vi "nano-positioner.vi"() -> ()   [LabVIEW 2014]
uses:
  <vilib>/Utility/inputDevices.llb/keyboardAcquire.vi
  <userlib>/Madlib/Madlib.dll
panel:
  in  "?":bool
  in  "Motion Multiplier":dbl(slide)=1.0 scale=1.0..100.0
  in  "Command rate":u16(ring)=10 items=["500 Hertz"=2, "100 Hertz"=10, "10 Hertz"=100, "1 Hertz"=1000]
  out "First Key":T1(ring)
  in  "Max Velocity":string(combo)="22"
  in  "Z Decreasing":string(combo)="21"
  in  "Z Increasing":string(combo)="24"
  in  "X Increasing":string(combo)="32"
  in  "X Decreasing":string(combo)="28"
  in  "Y Decreasing":string(combo)="10"
  in  "Y Increasing":string(combo)="13"
  out "Z (mM)":dbl format="%#_13g"
  out "Y (mM)":dbl format="%#_13g"
  out "X (mM)":dbl format="%#_13g"
  out "Z Range (mM)":dbl format="%#_13g"
  out "Y Range (mM)":dbl format="%#_13g"
  out "X Range (mM)":dbl format="%#_13g"
  # "Key Configuration"
  # "Command Rate"
  # "Motion Multiplier"
  # "x1"
  # "x100"
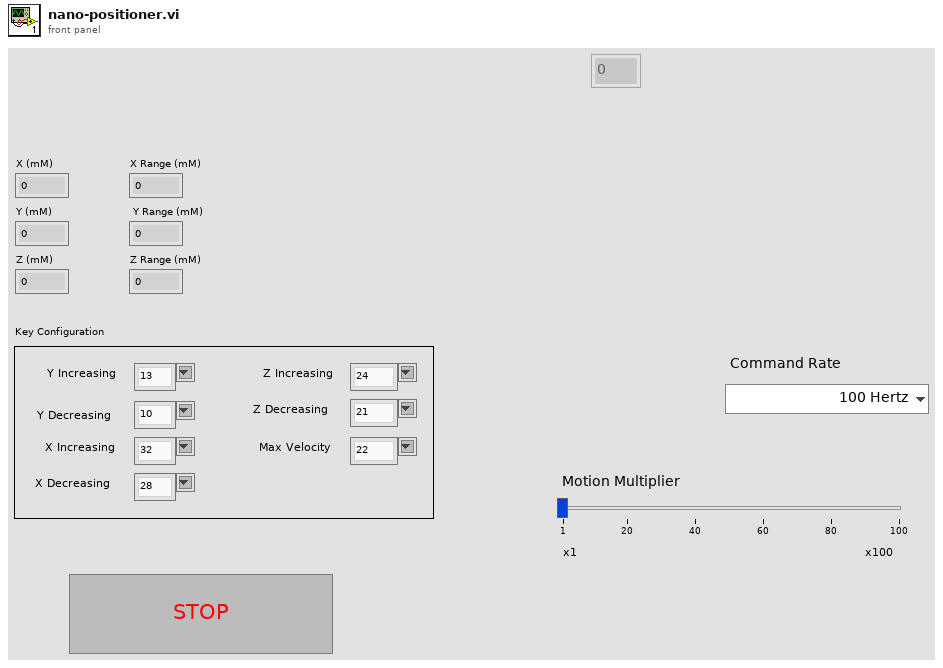
[diagram p1: front panel]
types:
  T1 = enum16{"0", "1", "2", "3", "4", "5", "6", "7", "8", "9", "A", "B", "C", "D", "E", "F", "G", "H", "I", "J", "K", "L", "M", "N", "O", "P", "Q", "R", "S", "T", "U", "V", "W", "X", "Y", "Z", "F1", "F2", "F3", "F4", "F5", "F6", "F7", "F8", "F9", "F10", "F11", "F12", "F13", "F14", "F15", "ADD", "BACK", "BACKSLASH", "CAPITAL", "COMMA", "DECIMAL", "DELETE", "DIVIDE", "DOWN", "END", "EQUALS", "ESCAPE", "GRAVE (`)", "HOME", "INSERT", "LBRACKET", "LCONTROL", "LEFT", "L ALT", "LSHIFT", "LWIN", "MINUS", "MULTIPLY", "NEXT", "NUMLOCK", "NUMPAD_0", "NUMPAD_1", "NUMPAD_2", "NUMPAD_3", "NUMPAD_4", "NUMPAD_5", "NUMPAD_6", "NUMPAD_7", "NUMPAD_8", "NUMPAD_9", "PAUSE", "PERIOD", "PRIOR (PG UP)", "RBRACKET", "RCONTROL", "RETURN", "RIGHT", "R ALT", "RSHIFT", "RWIN", "SCROLL", "SEMICOLON", "SLASH", "SPACE", "SUBTRACT", "TAB", "UP", "ENTER (num pad)", "' (quote)"}
  T2 = cluster{"X Command":dbl, "Y Command":dbl, "Z Command":dbl, "X Position":dbl, "Y Position":dbl, "Z Position":dbl, "X Calibration":dbl, "Y Calibration":dbl, "Z Calibration":dbl}
  T3 = cluster{"X Command":dbl, "Y Command":dbl, "Z Command":dbl, "X Position":dbl, "Y Position":dbl, "Z Position":dbl}
  T4 = enum16{"0", "1", "2", "3", "4", "5", "6", "7", "8", "9", "A", "B", "C", "D", "E", "F", "G", "H", "I", "J", "K", "L", "M", "N", "O", "P", "Q", "R", "S", "T", "U", "V", "W", "X", "Y", "Z", "F1", "F2", "F3", "F4", "F5", "F6", "F7", "F8", "F9", "F10", "F11", "F12", "F13", "F14", "F15", "ADD", "BACK", "BACKSLASH", "CAPITAL", "COMMA", "DECIMAL", "DELETE", "DIVIDE", "DOWN", "END", "EQUALS", "ESCAPE", "GRAVE (`)", "HOME", "INSERT", "LBRACKET", "LCONTROL", "LEFT", "L ALT", "LSHIFT", "LWIN", "MINUS", "MULTIPLY", "NEXT", "NUMLOCK", "NUMPAD_0", "NUMPAD_1", "NUMPAD_2", "NUMPAD_3", "NUMPAD_4", "NUMPAD_5", "NUMPAD_6", "NUMPAD_7", "NUMPAD_8", "NUMPAD_9", "PAUSE", "PERIOD", "PRIOR (PG UP)", "RBRACKET", "RCONTROL", "RETURN", "RIGHT", "R ALT", "RSHIFT", "RWIN", "SCROLL", "SEMICOLON", "SLASH", "SPACE", "SUBTRACT", "TAB", "UP", "ENTER (num pad)", "' (quote)"}[]
  T5 = cluster{"Y Increasing":string, "Y Decreasing":string, "X Increasing":string, "X Decreasing":string, "Z Increasing":string, "Z Decreasing":string, "Max Velocity":string}
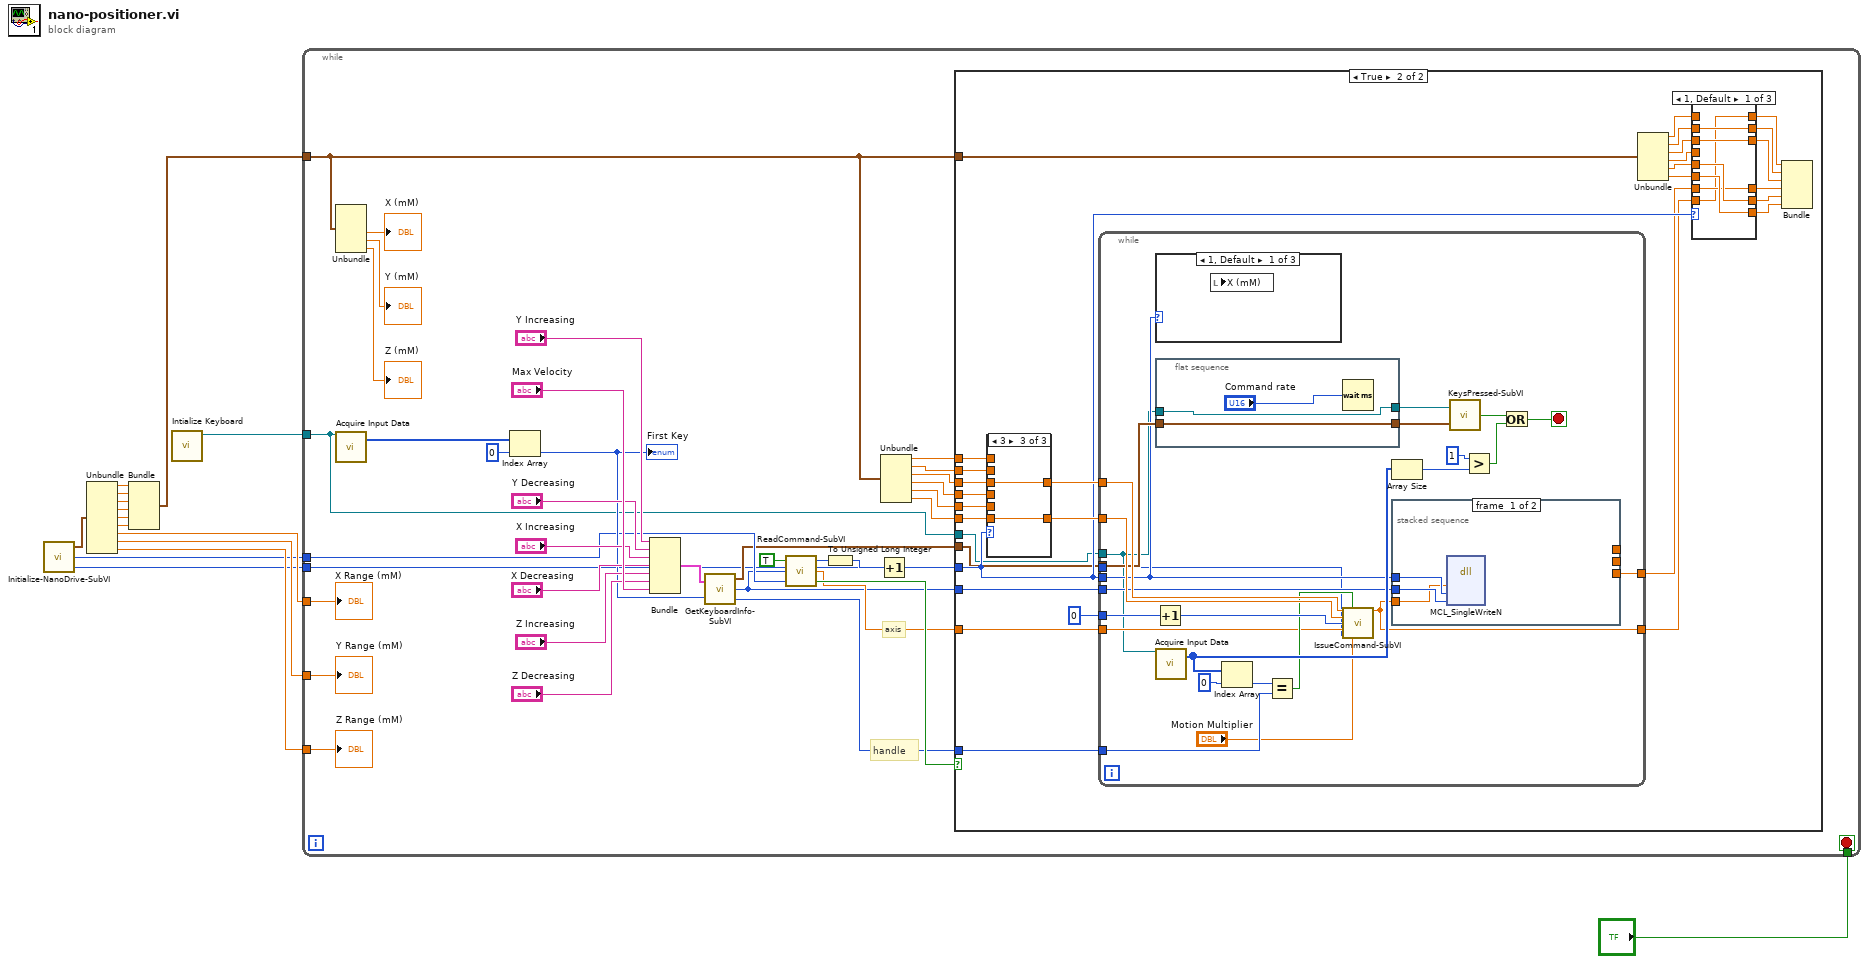
[diagram p0: block diagram]
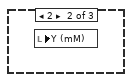
[diagram p5: hidden frame]
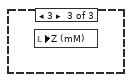
[diagram p6: hidden frame]
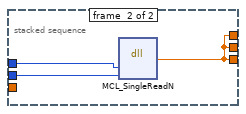
[diagram p7: hidden frame]
diagram:
  n1 = call <userlib>:"Initialize-NanoDrive-SubVI.vi"() -> ("Output Pos Info"=w15:T2, "Handle"=w3:i32, "ADC/DAC Resolution"=w2:u32)  [unwired: 1 in]
  n2 = Unbundle(w15) -> ("X Command"=w11:dbl, "Y Command"=w10:dbl, "Z Command"=w9:dbl, "X Position"=w8:dbl, "Y Position"=w7:dbl, "Z Position"=w6:dbl, "X Calibration"=w14:dbl, "Y Calibration"=w13:dbl, "Z Calibration"=w12:dbl)
  n3 = Bundle("X Command"=w11, "Y Command"=w10, "Z Command"=w9, "X Position"=w8, "Y Position"=w7, "Z Position"=w6) -> (w5:T3)  [unwired: 1 in]
  n4 = call <vilib>:"Intialize Keyboard.vi"() -> ("device ID"=w4:refnum<k1>)  [unwired: 1 in, 10 out]
  n5 = while {
    tunnel: w14 -> [w52]
    tunnel: w13 -> [w51]
    tunnel: w12 -> [w50]
    tunnel: w5 -> [w46]
    tunnel: w4 -> [w19]
    tunnel: w3 -> [w33]
    tunnel: w2 -> [w17]
    tunnel: "?" -> [w16]
    stop <- w16 stop-if-true
    # "handle"
    # "axis"
    n6 = Unbundle(w46) -> ("X Position"=→"X (mM)":dbl, "Y Position"=→"Y (mM)":dbl, "Z Position"=→"Z (mM)":dbl)  [unwired: 3 out]
    n7 = call-poly <vilib>:"Acquire Input Data.vi"("device ID"=w19) -> ("keys pressed"=w37:T4)  [unwired: 1 in, 17 out]
    n8 = Index Array "Index Array"(array=w37, index=0) -> (element=w35:T1)
    "First Key" <- w35
    n9 = Bundle("Y Increasing"="Y Increasing", "Y Decreasing"="Y Decreasing", "X Increasing"="X Increasing", "X Decreasing"="X Decreasing", "Z Increasing"="Z Increasing", "Z Decreasing"="Z Decreasing", "Max Velocity"="Max Velocity") -> (w38:T5)  [unwired: 1 in]
    n10 = call <userlib>:"GetKeyboardInfo-SubVI.vi"("Key Selections"=w38, "Key\nValue"=w35) -> ("Key values"=w20:cluster{i32, i32, i32, i32, i32, i32, i32}, "number"=w18:u32, "Max Velocity Value"=w22:i32)
    n11 = call <userlib>:"ReadCommand-SubVI.vi"("handle"=w33, "Motion #"=w18, "Enable\n(True)"=TRUE) -> ("Enable Move\n(TRUE)"=w32:bool, "Direction"=w21:dbl, "Axis"=w31:enum16{"X", "Y", "Z"})
    n12 = To Unsigned Long Integer(number=w31) -> (unsigned 32bit integer=w30:u32)
    n13 = Increment(x=w30) -> (x+1=w29:u32)
    n14 = Unbundle(w46) -> ("X Command"=w27:dbl, "Y Command"=w26:dbl, "Z Command"=w24:dbl, "X Position"=w28:dbl, "Y Position"=w25:dbl, "Z Position"=w23:dbl)
    n15 = case shown="True" w32 {
      tunnel: w46 -> [_ w83]
      tunnel: w29 -> [_ w61]
      tunnel: w28 -> [_ w82]
      tunnel: w27 -> [_ w81]
      tunnel: w26 -> [_ w78]
      tunnel: w25 -> [_ w77]
      tunnel: w24 -> [_ w76]
      tunnel: w23 -> [_ w75]
      tunnel: w22 -> [_ w60]
      tunnel: w21 -> [_ w59]
      tunnel: w20 -> [_ w58]
      tunnel: w19 -> [_ w57]
      tunnel: w18 -> [_ w56]
      tunnel: w17 -> [_ w53]
      frame False {
      }
      frame True {
        n16 = case shown="3" w61 {
          tunnel: [w85 w86 w88] -> w79
          tunnel: w82 -> [w85 _ _]
          tunnel: w81 -> [w84 _ _]
          tunnel: [w84 w87 w89] -> w80
          tunnel: w78 -> [_ w87 _]
          tunnel: w77 -> [_ w86 _]
          tunnel: w76 -> [_ _ w89]
          tunnel: w75 -> [_ _ w88]
          frame 1, Default {
          }
          frame 2 {
          }
          frame 3 {
          }
        }
        n17 = while {
          tunnel: w80 -> [w114]
          tunnel: w79 -> [w113]
          tunnel: 0 -> [w112]
          tunnel: w61 -> [w94]
          tunnel: w60 -> [w106]
          tunnel: w59 -> [w105]
          tunnel: w58 -> [w102]
          tunnel: w57 -> [w91]
          tunnel: w56 -> [w95]
          tunnel: [w93] -> w55
          tunnel: [w92] -> w54
          tunnel: w53 -> [w90]
          stop <- w96 stop-if-true
          n18 = Increment(x=w112) -> (x+1=w111:i32)
          n19 = case shown="1, Default" w94 {
            frame 1, Default {
              n20 = local read "X (mM)"() -> ()  [unwired: 1 in]
            }
            frame 2 {
              n21 = local read "Y (mM)"() -> ()  [unwired: 1 in]
            }
            frame 3 {
              n22 = local read "Z (mM)"() -> ()  [unwired: 1 in]
            }
          }
          n23 = flat-sequence {
            tunnel: [w122] -> w104
            tunnel: w91 -> [w122]
            tunnel: [w121] -> w103
            tunnel: w102 -> [w121]
            frame #0 {
              n24 = Wait (ms)(milliseconds to wait="Command rate") -> ()  [unwired: 1 out]
            }
          }
          n25 = call-poly <vilib>:"Acquire Input Data.vi"("device ID"=w91) -> ("keys pressed"=w109:T4)  [unwired: 1 in, 17 out]
          n26 = Index Array(array=w109, index=0) -> (element=w108:T1)
          n27 = Equal?(x=w108, y=w106) -> (x = y?=w107:bool)
          n28 = call <userlib>:"IssueCommand-SubVI.vi"("Current Position"=w114, "Max Velocity?"=w107, "Calibration"=w113, "Loop Iteration"=w111, "Direction"=w105, "ADC/DAC Resolution"=w90, "Motion Multiplier"="Motion Multiplier") -> ("Pos. Command"=w92:dbl)  [unwired: 7 in, 1 out]
          n29 = Array Size(array=w109) -> (size(s)=w100:i32)
          n30 = stacked-sequence {
            tunnel: w95 -> [w117 w119]
            tunnel: w94 -> [w116 w120]
            tunnel: [_ w118] -> _
            tunnel: w92 -> [w115 _]
            tunnel: [_ w118] -> _
            tunnel: [_ w118] -> w93
            frame #0 {
              n31 = dll-call lib="C:/Program Files (x86)/National Instruments/LabVIEW 2014/user.lib/Madlib/Madlib.dll" fn="MCL_SingleWriteN" label="Madlib.dll\nMCL_SingWriteN"("position"=w115, "axis"=w116, "handle"=w117) -> ()  [unwired: 6 in, 3 out]
            }
            frame #1 {
              n32 = dll-call lib="C:/Program Files (x86)/National Instruments/LabVIEW 2014/user.lib/Madlib/Madlib.dll" fn="MCL_SingleReadN" label="Madlib.dll:\nMCL_SingleReadN"("Axis"=w120, "Handle"=w119) -> ("position"=w118:dbl)  [unwired: 5 in, 2 out]
            }
          }
          n33 = call <userlib>:"KeysPressed-SubVI.vi"("Key values"=w103, "device ID"=w104) -> ("Stop = TRUE"=w98:bool)
          n34 = Greater?(x=1, y=w100) -> (0:w97:bool)
          n35 = Or(x=w98, y=w97) -> (x .or. y?=w96:bool)
        }
        n36 = Unbundle(w83) -> ("X Command"=w74:dbl, "Y Command"=w73:dbl, "Z Command"=w72:dbl, "X Position"=w71:dbl, "Y Position"=w70:dbl, "Z Position"=w69:dbl)
        n37 = case shown="1, Default" w61 {
          tunnel: w74 -> [_ w135 w141]
          tunnel: w73 -> [w129 _ w140]
          tunnel: w72 -> [w128 w133 _]
          tunnel: w71 -> [_ w134 w139]
          tunnel: w70 -> [w127 _ w138]
          tunnel: w69 -> [w126 w132 _]
          tunnel: [w129 w130 w140] -> w68
          tunnel: [w128 w133 w136] -> w67
          tunnel: [w127 w131 w138] -> w65
          tunnel: [w126 w132 w137] -> w66
          tunnel: [w124 w135 w141] -> w64
          tunnel: [w125 w134 w139] -> w63
          tunnel: w55 -> [w125 w131 w137]
          tunnel: w54 -> [w124 w130 w136]
          frame 1, Default {
          }
          frame 2 {
          }
          frame 3 {
          }
        }
        n38 = Bundle("X Command"=w64, "Y Command"=w68, "Pos. Command"=w67, "X Position"=w63, "Y Position"=w65, "position"=w66) -> ()  [unwired: 1 in, 1 out]
      }
    }
    "X Range (mM)" <- w52
    "Y Range (mM)" <- w51
    "Z Range (mM)" <- w50
  }
